vi "sedSpectrometer_getEvent_Timeout.vi"(8 "error in (no error)":errorcluster, 11 "logevent_Timeout_Ctl":T1) -> (0 "error out":errorcluster, 2 "function return":i32, 3 "logevent_Timeout_Ctl out":T1)   [LabVIEW 2016, in "SALLV_sedSpectrometer.lvlib"]
doc: "int sedSpectrometer_shm_getEvent_TimeoutLV(sedSpectrometer_logevent_TimeoutLV *logevent_Timeout_Ctl );"
uses:
  SALLV_sedSpectrometer.lvlib
  DataTypes/logevent_Timeout.ctl
  SALLV_sedSpectrometer.so
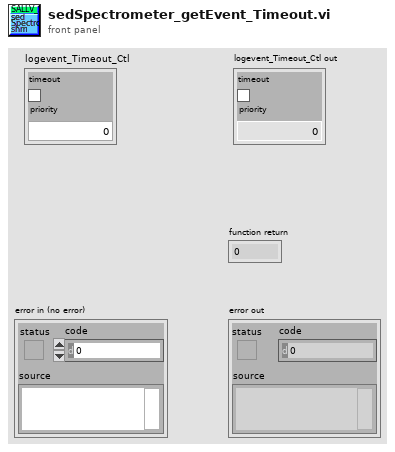
[diagram p1: front panel]
types:
  T1 = typedef "SALLV_sedSpectrometer.lvlib/logevent_Timeout.ctl" = cluster{"timeout":bool, "priority":i32}
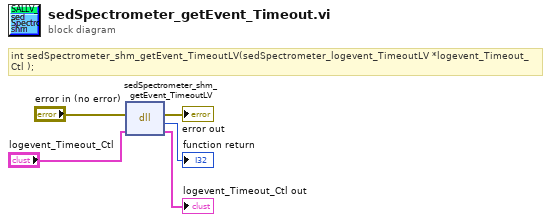
[diagram p0: block diagram]
diagram:
  # "int sedSpectrometer_shm_getEvent_TimeoutLV(sedSpectrometer_logevent_TimeoutLV *logevent_Timeout_Ctl );"
  n1 = dll-call lib="home/harini/TCS/SALLV_sedSpectrometer/SALLV_sedSpectrometer.*" fn="sedSpectrometer_shm_getEvent_TimeoutLV"(error in="error in (no error)", "logevent_Timeout_Ctl"="logevent_Timeout_Ctl") -> (error out=→"error out":errorcluster, →"function return":i32, "logevent_Timeout_Ctl"=→"logevent_Timeout_Ctl out":T1)  [unwired: 2 in, 1 out]
